vi "Calibration Engine (global).vi"(0 "Calibrated In":bool, 2 "Mode":T1(ring), 5 "Load File In":bool, 7 "Version In":string, 11 "Error In":errorcluster) -> (4 "Calibrated Out":bool, 6 "Load File Out":bool, 8 "Version Out":string, 10 "File Loaded":bool, 14 "Engine Error Count":i32, 15 "Error Out":errorcluster)   [LabVIEW 2013]
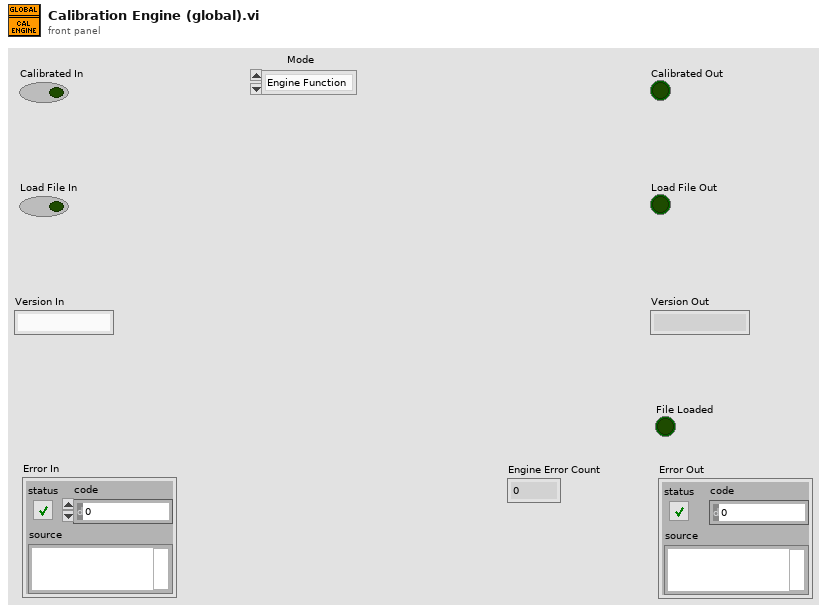
[diagram p1: front panel]
types:
  T1 = enum16{"Engine Function", "Read Version", "Read Calibrated", "Read Load File", "Confirm File", "Read Confirmation", "Cal Engine Errors"}
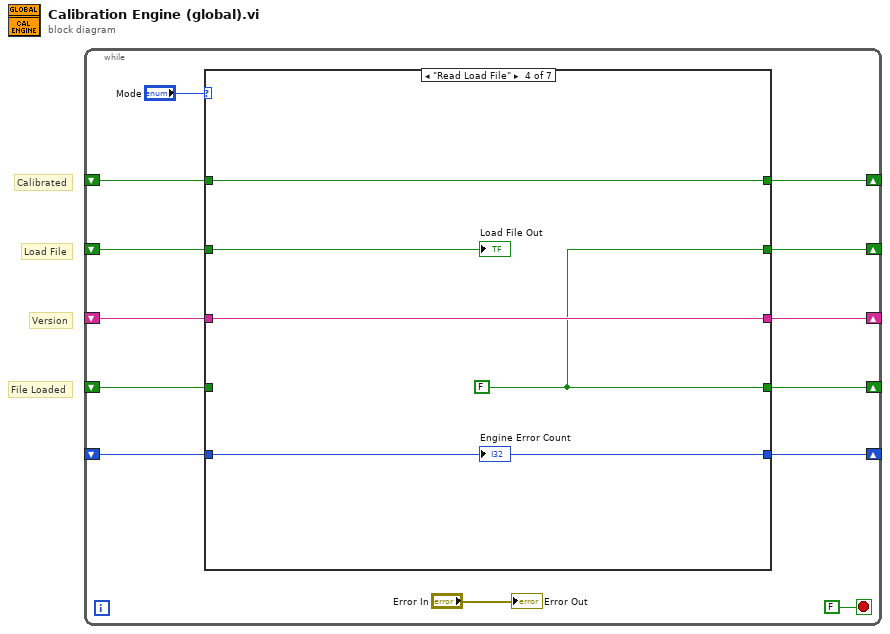
[diagram p0: block diagram]
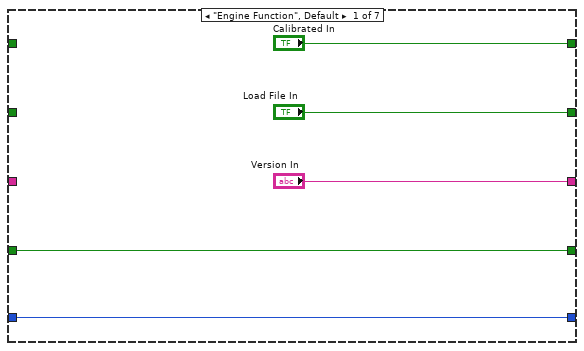
[diagram p2: hidden frame]
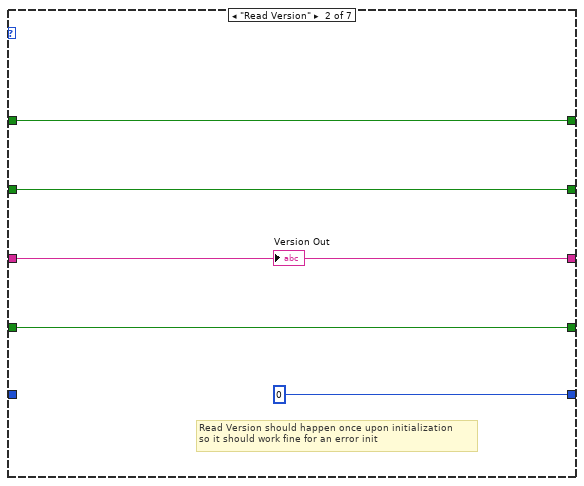
[diagram p3: hidden frame]
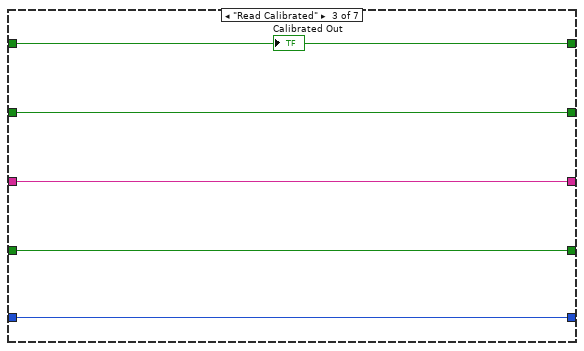
[diagram p4: hidden frame]
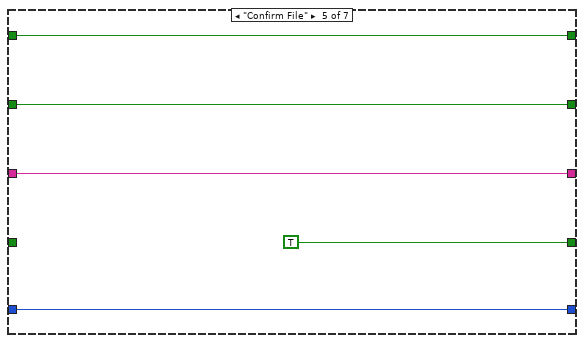
[diagram p5: hidden frame]
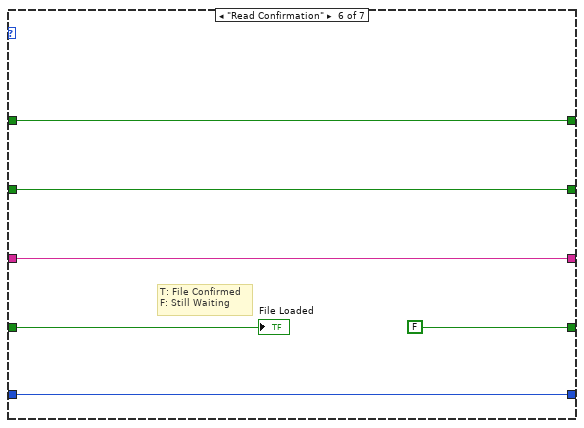
[diagram p6: hidden frame]
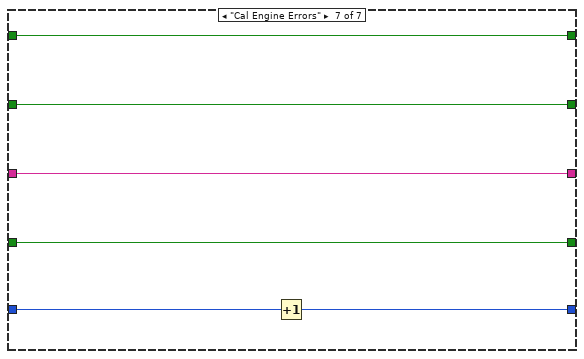
[diagram p7: hidden frame]
diagram:
  # "File Loaded"
  # "Version"
  # "Load File"
  # "Calibrated"
  n1 = while {
    shift-right: [w11] -> _
    shift-left: _ -> [w8]
    shift-right: [w10] -> _
    shift-left: _ -> [w7]
    shift-right: [w9] -> _
    shift-left: _ -> [w6]
    shift-right: [w5] -> _
    shift-left: _ -> [w4]
    shift-right: [w2] -> _
    shift-left: _ -> [w1]
    stop <- FALSE stop-if-true
    n2 = case shown="\"Read Load File\"" "Mode" {
      tunnel: ["Calibrated In" w23 w28 w33 w36 w42 w50] -> w11
      tunnel: ["Load File In" w22 w27 w29 w35 w43 w49] -> w10
      tunnel: ["Version In" w21 w26 w31 w37 w44 w48] -> w9
      tunnel: w8 -> [_ w23 w28 w33 w36 w42 w50]
      tunnel: w7 -> [_ w22 w27 w32 w35 w43 w49]
      tunnel: w6 -> [_ w21 w26 w31 w37 w44 w48]
      tunnel: [w15 w20 w25 w29 TRUE FALSE ("t") w47] -> w5
      tunnel: w4 -> [w15 w20 w25 _ _ w41 w47]
      tunnel: [w14 0 w24 w30 w34 w39 w45] -> w2
      tunnel: w1 -> [w14 _ w24 w30 w34 w39 w46]
      frame "Engine Function", Default {
      }
      frame "Read Version" {
        # "Read Version should happen once upon initialization\nso it should work fine for an error init"
        "Version Out" <- w21
      }
      frame "Read Calibrated" {
        "Calibrated Out" <- w28
      }
      frame "Read Load File" {
        w29 = FALSE
        "Load File Out" <- w32
        "Engine Error Count" <- w30
      }
      frame "Confirm File" {
      }
      frame "Read Confirmation" {
        # "T: File Confirmed\nF: Still Waiting"
        "File Loaded" <- w41
      }
      frame "Cal Engine Errors" {
        n3 = Increment(x=w46) -> (x+1=w45:i32)
      }
    }
    "Error Out" <- "Error In"
  }
